vi "PH_Beamline.set 6P Switch State in GUI.vi"(0 "i ref in":refnum<vi>, 1 "Boolean GUI Ref":refnum<vi>, 2 "Picture GUI Ref":refnum<vi>, 3 "Status":T1 items=["no info", "off/false/out", "on/true/in", "Failure", "Alarm", "Status 1", "Status 2", "Status 3"], 4 "no Link?":bool, 5 "error in":errorcluster) -> (14 "i ref out":refnum<vi>, 19 "error out":errorcluster)   [LabVIEW 2014, in "PH_Beamline.lvlib"]
doc: "This VI sets the 6P Switch State GUI object."
uses:
  PH_Beamline.lvlib
  PH_Basics/PH_StatusHandler/PH_StatusHandler.Status.ctl
  PH_BL-Master/PH_BL-Master.Shutter State.ctl
  PH_Basics/PH_Common/PH_Common.lvlib
  PH_BL-Master/PH_BL-Master.lvlib
  PH_Basics/PH_StatusHandler/PH_StatusHandler.lvlib
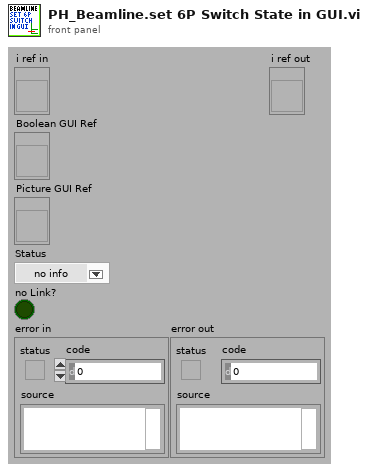
[diagram p1: front panel]
types:
  T1 = typedef "PH_StatusHandler.lvlib/PH_StatusHandler.Status.ctl" = i16
  T2 = typedef "PH_BL-Master.lvlib/PH_BL-Master.Shutter State.ctl" = enum16{"No Link", "No Info", "In", "Out", "in between"}
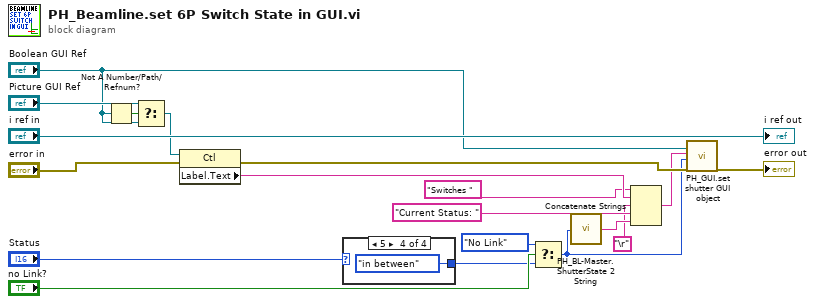
[diagram p0: block diagram]
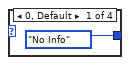
[diagram p2: hidden frame]
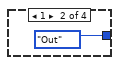
[diagram p3: hidden frame]
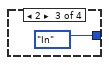
[diagram p4: hidden frame]
diagram:
  n1 = Not A Number/Path/Refnum?(number/path/refnum="Boolean GUI Ref") -> (NaN/Path/Refnum?=w11:bool)
  n2 = Select(t="Picture GUI Ref", s=w11, f="Boolean GUI Ref") -> (s? t:f=w13:refnum<vi>)
  n3 = property class="Ctl"(reference=w13, error in="error in") -> (error out=w15:errorcluster, "Label.Text"=w10:string)  [unwired: 1 out]
  n4 = case shown="5" "Status" {
    tunnel: [PH_BL-Master.Shutter_State."No Info" ("Shutter State") PH_BL-Master.Shutter_State."Out" ("Shutter State") PH_BL-Master.Shutter_State."In" ("Shutter State") PH_BL-Master.Shutter_State."in between" ("Shutter State")] -> w8
    frame 0, Default {
    }
    frame 1 {
    }
    frame 2 {
    }
    frame 5 {
    }
  }
  n5 = Select(t=PH_BL-Master.Shutter_State."No Link" ("Shutter State"), s="no Link?", f=w8) -> (s? t:f=w3:T2)
  n6 = call "PH_BL-Master.ShutterState 2 String.vi"("Shutter State"=w3) -> ("String"=w2:string)
  n7 = Concatenate Strings("Switches " ("string"), w10, "\r", "Current Status: " ("string"), w2) -> (w4:string)
  n8 = call "PH_GUI.set shutter GUI object.vi"("Wanted Boolean Ref"="Boolean GUI Ref", "Tip Strip"=w4, "Shutter State"=w3, "error in (no error)"=w15) -> ("error out"=→"error out":errorcluster)  [unwired: 15 in]
  "i ref out" <- "i ref in"
